vi "WinCI Set HWND.vi"(8 "error in (no error)":errorcluster, 9 "use active window? (F)":bool, 10 "window handle":i32) -> (0 "error out":errorcluster)   [LabVIEW 2017, in "NI_SCC_WinCI.lvlib"]
uses:
  <vilib>/SourceControl/Providers/WinCI/NI_SCC_WinCI.lvlib
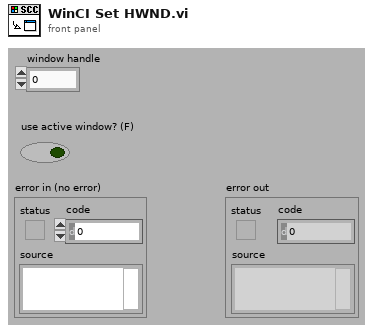
[diagram p1: front panel]
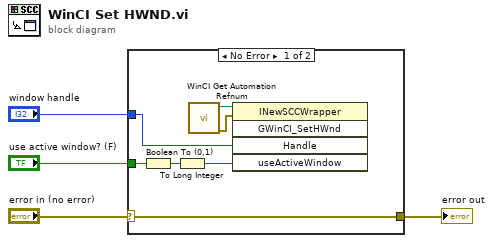
[diagram p0: block diagram]
diagram:
  n1 = case shown="No Error" "error in (no error)" {
    selector: "error in (no error)" -> [w11 w12]
    tunnel: [w11 w12] -> w3
    tunnel: "use active window? (F)" -> [w9 _]
    tunnel: "window handle" -> [w8 _]
    frame No Error {
      n2 = Boolean To (0,1)(Boolean=w9) -> (0, 1=w10:i16)
      n3 = To Long Integer(number=w10) -> (32bit integer=w7:i32)
      n4 = call <vilib>:"WinCI Get Automation Refnum.vi"() -> ("error out"=w6:errorcluster, "automation refnum"=w5:refnum<k7>)  [unwired: 10 out]
      n5 = invoke class="INewSCCWrapper" method="GWinCI_SetHWnd"(reference=w5, error in=w6, "Handle"=w8, "useActiveWindow"=w7) -> ()  [unwired: 1 in, 5 out]
    }
    frame Error {
    }
  }
  "error out" <- w3
